vi "KH TURCK ETHERNETIP RFID ST READ Global.vi"() -> ()   [LabVIEW 2021]
uses:
  KH TURCK ETHERNETIP TDef Enum RFID Data RFID.ctl
panel:
  out "RFID 0 Read SM":T1[](array[typedef])
  out "RFID 1 Read SM":T1[](array[typedef])
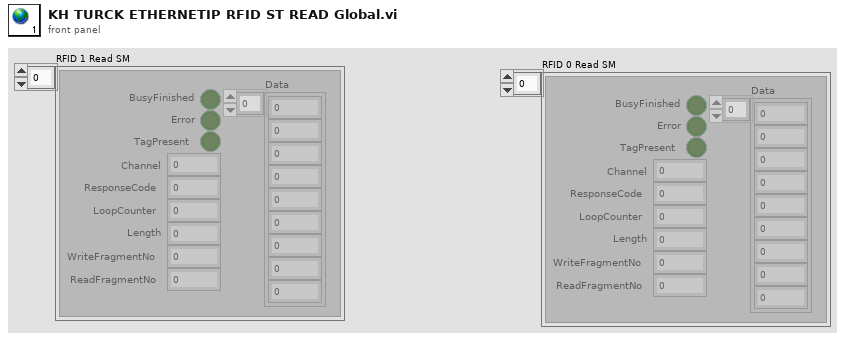
[diagram p1: front panel]
types:
  T1 = typedef "KH TURCK ETHERNETIP TDef Enum RFID Data RFID.ctl" = cluster{"ResponseCode":u16, "LoopCounter":u8, "Length":u16, "WriteFragmentNo":u8, "ReadFragmentNo":u8, "Data":u8[], "TagPresent":bool, "Error":bool, "BusyFinished":bool, "Channel":u16}
diagram:
